vi "Set Bliley Relay - Fast2023.vi"(1 "Data Position":u8=1 min=1 max=8, 2 "RF Position":u8=1 min=1 max=63 step=1, 3 "error in":errorcluster, 4 "GPIB Address":u8=16 min=1 max=31, 5 "System Number":u8=1 min=1 max=5) -> (0 "error out":errorcluster)   [LabVIEW 2023]
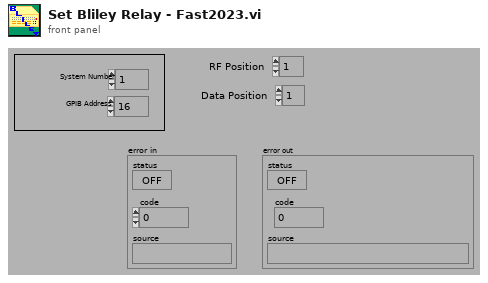
[diagram p1: front panel]
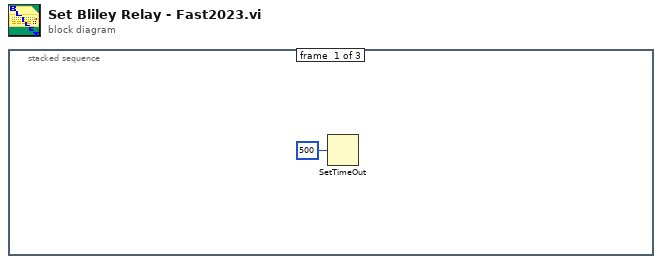
[diagram p0: block diagram]
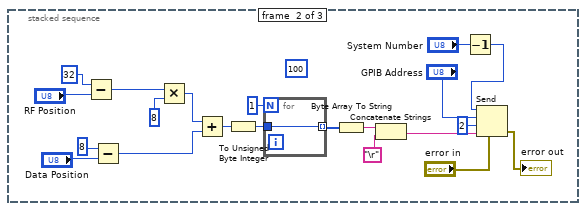
[diagram p2: hidden frame]
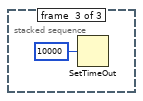
[diagram p3: hidden frame]
diagram:
  n1 = stacked-sequence {
    frame #0 {
      n2 = SetTimeOut(1:500 ("new timeout (10000)")) -> ()  [unwired: 1 out]
    }
    frame #1 {
      (unwired) 100 ("timeout ms (488.2 global)")
      n3 = Subtract(x=u8 32 ("y"), y="RF Position") -> (x-y=w5:u8)
      n4 = Subtract(x=u8 8 ("y"), y="Data Position") -> (x-y=w6:u8)
      n5 = Multiply(x=w5, y=i16 8) -> (x*y=w21:i16)
      n6 = Add(x=w21, y=w6) -> (x+y=w20:i16)
      n7 = To Unsigned Byte Integer(number=w20) -> (unsigned 8bit integer=w14:u8)
      n8 = for {
        N: 1 -> [_]
        tunnel: [w23] -> w13 mode=indexing
        tunnel: w14 -> [w23]
      }
      n9 = Byte Array To String(unsigned byte array=w13) -> (string=w15:string)
      n10 = Concatenate Strings(w15, "\r") -> (w12:string)
      n11 = Decrement(x="System Number") -> (x-1=w9:u8)
      n12 = Send(0:w9, 2:"GPIB Address", 3:i16 2 ("mode"), 4:"error in", 5:w12) -> (8:→"error out":errorcluster)  [unwired: 2 out]
    }
    frame #2 {
      n13 = SetTimeOut(1:10000 ("new timeout (10000)")) -> ()  [unwired: 1 out]
    }
  }
